vi "MainProgrammer.vi"() -> ()   [LabVIEW 2017]
uses:
  <vilib>/Instr/_visa.llb/Select Event Type.ctl
  <vilib>/Utility/config.llb/Read Key (String).vi
  <vilib>/Utility/config.llb/Write Key (String).vi
  <vilib>/Instr/_visa.llb/VISA Configure Serial Port (Instr).vi
  <vilib>/Utility/config.llb/NI_LVConfig.lvlib
panel:
  out "read buffer":string
  out "Rx":u64
  out "Tx":u64
  in  "stop 7":bool
  in  "stop 6":bool
  out "Error List":string
  out "COM Port":bool
  in  "Flash Baud":u32(ring)=115200 caption="Flash Baudrate" items=["4800"=4800, "9600"=9600, "19200"=19200, "38400"=38400, "57600"=57600, "115200"=115200, "230400"=230400, "460800"=460800, "921600"=921600]
  in  "cmd Baud":u32(ring)=230400 items=["4800"=4800, "9600"=9600, "19200"=19200, "38400"=38400, "57600"=57600, "115200"=115200, "230400"=230400, "460800"=460800, "921600"=921600]
  in  "COM Port":refnum<visa-resource-name>="COM4"
  in  "Next Button":bool
  in  "File Path Control":path
  out "CheckSumArray":u16[][](array[numeric]) format="%.0x"
  out "CheckSum DataB":u16 format="%.0x"
  out "CheckSum Data":u16 format="%.0x"
  out "Array 3":u16[][](array[numeric]) format="%.0x"
  out "Num of Data packet":i32
  out "sumHeader":u16 format="%.0x"
  out "error out":errorcluster
  # "Ver 1.0.5"
  # "© Redler Technologies. All Rights Reserved"
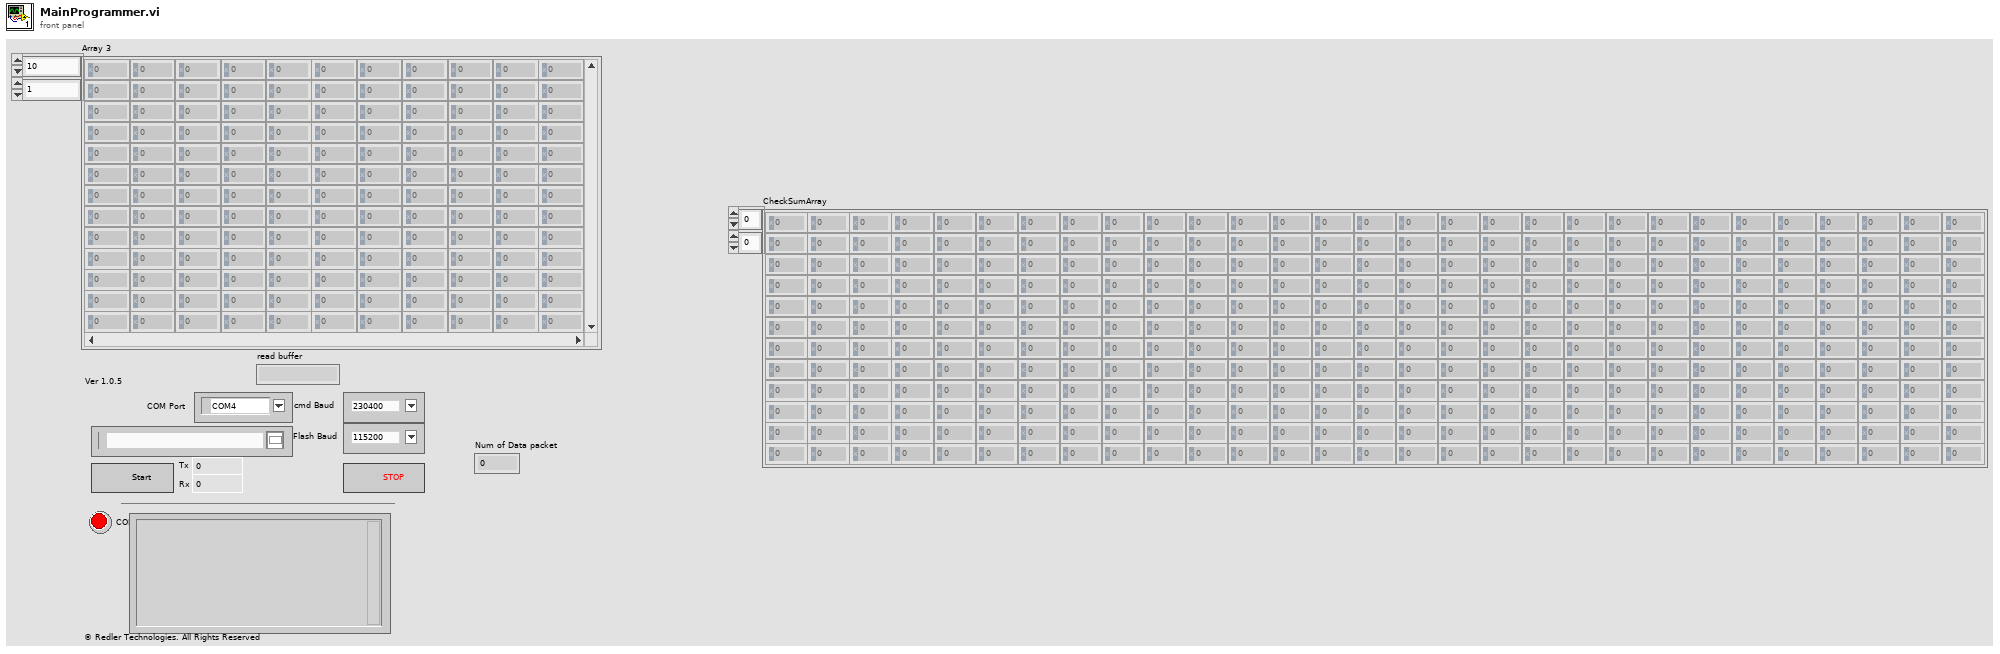
[diagram p1: front panel]
types:
  T1 = typedef "NI_LVConfig.lvlib/Config Data RefNum.ctl" = refnum<k1>
  T2 = cluster{"Send Debug":string, "idx":u16, "DataType":enum8{"Int", " float"}, "Cmd id":u16, "Get/Set":enum8{"Set", "Get"}}
  T3 = cluster{"Data":string, "idx":u16, "DataType":enum8{"Int", " float"}, "Cmd id":u16, "Get/Set":enum8{"Set", "Get"}}
  T4 = typedef "Select Event Type.ctl" = u32
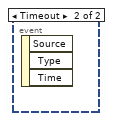
[diagram p3: hidden frame]
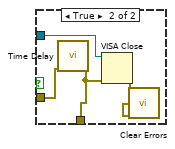
[diagram p4: hidden frame]
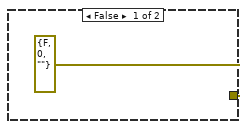
[diagram p5: hidden frame]
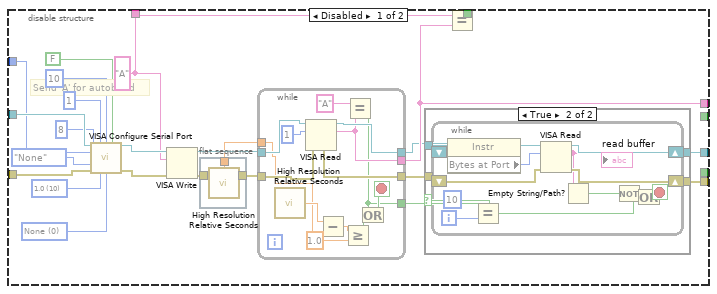
[diagram p7: hidden frame]
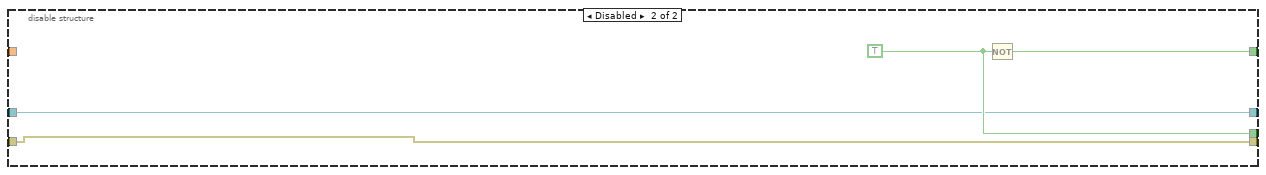
[diagram p10: hidden frame]
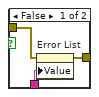
[diagram p13: hidden frame]
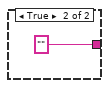
[diagram p16: hidden frame]
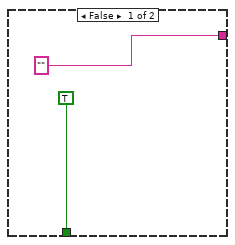
[diagram p17: hidden frame]
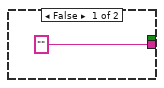
[diagram p18: hidden frame]
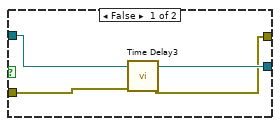
[diagram p19: hidden frame]
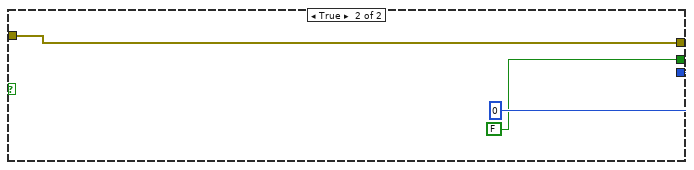
[diagram p20: hidden frame]
diagram:
  w8 = u32 230400 items=["4800"=4800, "9600"=9600, "19200"=19200, "38400"=38400, "57600"=57600, "115200"=115200, "230400"=230400, "460800"=460800, "921600"=921600] ("cmd Baud")
  w9 = u32 230400 items=["4800"=4800, "9600"=9600, "19200"=19200, "38400"=38400, "57600"=57600, "115200"=115200, "230400"=230400, "460800"=460800, "921600"=921600] ("Flash Baud")
  w18 = u32 230400 ("default (0 I32)")
  w3 = "Firmware Path" ("key")
  w4 = "Rayon" ("section")
  n1 = control-ref of="This VI"() -> (w39:refnum<vi>)
  n2 = invoke class="VI" method="Default Vals.Reinit All"(reference=w39, error in=errorcluster {"status"=FALSE, "code"=0, "source"=""} ("error in (no error)")) -> (error out=w7:errorcluster)  [unwired: 1 in, 2 out]
  n3 = property on="Flash Baud" class="Ring (strict)"(error in=w7, "Value"=w9) -> (error out=w10:errorcluster)  [unwired: 1 in, 1 out]
  n4 = property on="cmd Baud" class="Ring (strict)"(error in=w10, "Value"=w8) -> (error out=w6:errorcluster)  [unwired: 1 in, 1 out]
  n5 = call <vilib>:"Application Directory.vi"() -> ("Application Directory"=w37:path)
  n6 = Build Path(base path=w37, name or relative path="data\\RayonSerialProgramerConfigurationFile.ini") -> (appended path=w29:path)
  n7 = call <vilib>:"Open Config Data.vi"("error in (no error)"=w6, "create file if necessary (T)"=FALSE, "configuration file path"=w29) -> ("error out"=w33:errorcluster, "refnum"=w34:T1)  [unwired: 7 out]
  n8 = call-poly <vilib>:"Read Key.vi"("section"=w4, "error in (no error)"=w33, "key"=w3, "refnum"=w34) -> ("error out"=w1:errorcluster, "value"=w32:string, "refnum out"=w5:T1)  [unwired: 2 in, 3 out]
  n9 = String To Path(string=w32) -> (path=w31:path)
  n10 = property on="File Path Control" class="Path"(error in=w1, "Value"=w31) -> (error out=w2:errorcluster)  [unwired: 1 in, 1 out]
  n11 = call-poly <vilib>:"Read Key.vi"("section"=w4, "error in (no error)"=w2, "key"="COM", "refnum"=w5) -> ("error out"=w22:errorcluster, "value"=w14:string, "refnum out"=w27:T1)  [unwired: 2 in, 3 out]
  n12 = Type Cast(type=refnum<visa-resource-name> "COM1" ("UUT COM Port 2"), x=w14) -> (*(type *) &x=w13:refnum<visa-resource-name>)
  n13 = property on="COM Port" class="VISAName"("Value"=w13) -> ()  [unwired: 2 in, 2 out]
  n14 = call-poly <vilib>:"Read Key.vi"("section"=w4, "error in (no error)"=w22, "key"="Flash Baud", "refnum"=w27) -> ("error out"=w21:errorcluster, "value"=w20:string, "refnum out"=w28:T1)  [unwired: 2 in, 3 out]
  n15 = Decimal String To Number(string=w20, default (0L)=w18) -> (number=w16:u32)  [unwired: 1 in, 1 out]
  n16 = property on="Flash Baud" class="Ring (strict)"("Value"=w16) -> ()  [unwired: 2 in, 2 out]
  n17 = call-poly <vilib>:"Read Key.vi"("section"=w4, "error in (no error)"=w21, "key"="Boot Baud", "refnum"=w28) -> ("error out"=w11:errorcluster, "value"=w19:string, "refnum out"=w26:T1)  [unwired: 2 in, 3 out]
  n18 = Decimal String To Number(string=w19, default (0L)=w18) -> (number=w17:u32)  [unwired: 1 in, 1 out]
  n19 = property on="cmd Baud" class="Ring (strict)"("Value"=w17) -> ()  [unwired: 2 in, 2 out]
  n20 = call <vilib>:"Close Config Data.vi"("error in (no error)"=w11, "refnum"=w26) -> ("error out"=w12:errorcluster)  [unwired: 1 in, 8 out]
  n21 = while {
    tunnel: w12 -> [_]
    i -> [w41]
    stop <- w40 stop-if-true
    n22 = event shown="[0] \"stop 7\": Value Change" {
      selector: _ -> [_ _]
      dyn-events: _ -> [_ _]
      timeout: _ -> [_ _]
      tunnel: w41 -> [_ _]
      tunnel: [w42 _] -> w40
      event "stop 7": Value Change {
        n23 = event-data() -> ()  [unwired: 1 in, 3 out]
        n24 = Two Button Dialog(message="Are you sure to close? ", 1:"No" ("F button name (\"Cancel\")"), 2:"Yes" ("T button name (\"OK\")")) -> (T button?=w42:bool)
        n25 = property on="stop 6" class="Bool (strict)"("Value"=w42) -> (error out=w43:errorcluster)  [unwired: 2 in, 1 out]
        n26 = property on="stop 7" class="Bool (strict)"(error in=w43, "Value"=w42) -> (error out=w44:errorcluster)  [unwired: 1 in, 1 out]
        n27 = case shown="True" w42 {
          selector: w42 -> [_ w55]
          tunnel: w44 -> [_ w56]
          frame False {
          }
          frame True {
            w53 = "\r\n"
            n28 = property on="Error List" class="Str"(error in=w56) -> ("Value"=w49:string)  [unwired: 1 in, 2 out]
            n29 = Format Date/Time String(time format string (%c)="%H:%M:%S") -> (date/time string=w52:string)  [unwired: 2 in]
            n30 = Concatenate Strings(w52, " Operation stopped by user") -> (w48:string)
            n31 = Concatenate Strings(w48, w53, w49, w53) -> (w57:string)
            n32 = property on="Error List" class="Str"("Value"=w57) -> (error out=w54:errorcluster)  [unwired: 2 in, 1 out]
            n33 = flat-sequence {
              tunnel: w55 -> [_]
              tunnel: w54 -> [_]
              frame #0 {
                n34 = property on="stop 7" class="Bool (strict)"("Value"=FALSE ("stop 7")) -> ()  [unwired: 2 in, 2 out]
              }
            }
          }
        }
      }
      event Timeout {
        n35 = event-data() -> ()  [unwired: 1 in, 3 out]
      }
    }
  }
  n36 = while {
    tunnel: w12 -> [w67]
    tunnel: w4 -> [w94]
    tunnel: w3 -> [w93]
    tunnel: [w95] -> w30
    tunnel: w29 -> [w92]
    stop <- w62 stop-if-true
    w84 = FALSE ("Next Button")
    n37 = property on="File Path Control" class="Path"(error in=w67, "PTooLngToFt"=enum32{"Abbreviate Path", "Clip Path"}."Abbreviate Path" ("Path Too Long To Fit")) -> (error out=w59:errorcluster)  [unwired: 1 in, 1 out]
    n38 = property on="stop 6" class="Bool (strict)"(error in=w59, "Value"=FALSE ("stop 6")) -> (error out=w74:errorcluster)  [unwired: 1 in, 1 out]
    n39 = while {
      tunnel: ["COM Port"] -> w65
      tunnel: ["Flash Baud"] -> w103
      tunnel: ["cmd Baud"] -> w102
      tunnel: ["File Path Control"] -> w77
      tunnel: w94 -> [w984]
      tunnel: w74 -> [w980]
      tunnel: w93 -> [w982]
      tunnel: w92 -> [w978]
      tunnel: [w970] -> w66
      stop <- w981 stop-if-true
      n40 = call <vilib>:"Open Config Data.vi"("error in (no error)"=w980, "create file if necessary (T)"=FALSE, "configuration file path"=w978) -> ("error out"=w979:errorcluster, "refnum"=w976:T1)  [unwired: 7 out]
      n41 = Path To String(path="File Path Control") -> (string=w983:string)
      n42 = call <vilib>:"Is Path and Not Empty.vi"("path"="File Path Control") -> ("Is Path and Not Empty?"=w987:bool)  [unwired: 4 in]
      n43 = Not(x=w987) -> (.not. x?=w985:bool)
      n44 = And(x=w985, y="Next Button") -> (x .and. y?=w986:bool)
      n45 = case shown="False" w986 {
        tunnel: w984 -> [w996 _]
        tunnel: w979 -> [w1013 w1014]
        tunnel: w983 -> [w1012 _]
        tunnel: w982 -> [w1011 _]
        tunnel: w976 -> [w1010 _]
        tunnel: [w1009 w1015] -> w970
        tunnel: "COM Port" -> [w993 _]
        tunnel: "Flash Baud" -> [w990 _]
        tunnel: "cmd Baud" -> [w992 _]
        frame False {
          n46 = call-poly <vilib>:"Write Key.vi"("section"=w996, "error in (no error)"=w1013, "value"=w1012, "key"=w1011, "refnum"=w1010) -> ("error out"=w1003:errorcluster, "refnum out"=w999:T1)  [unwired: 1 in, 4 out]
          n47 = Type Cast(type="", x=w993) -> (*(type *) &x=w991:string)
          n48 = call-poly <vilib>:"Write Key.vi"("section"=w996, "error in (no error)"=w1003, "value"=w991, "key"="COM", "refnum"=w999) -> ("error out"=w1002:errorcluster, "refnum out"=w998:T1)  [unwired: 1 in, 4 out]
          n49 = Number To Decimal String(number=w990) -> (decimal integer string=w1008:string)  [unwired: 1 in]
          n50 = call-poly <vilib>:"Write Key.vi"("section"=w996, "error in (no error)"=w1002, "value"=w1008, "key"="Flash Baud", "refnum"=w998) -> ("error out"=w1001:errorcluster, "refnum out"=w997:T1)  [unwired: 1 in, 4 out]
          n51 = Number To Decimal String(number=w992) -> (decimal integer string=w1005:string)  [unwired: 1 in]
          n52 = call-poly <vilib>:"Write Key.vi"("section"=w996, "error in (no error)"=w1001, "value"=w1005, "key"="Boot Baud", "refnum"=w997) -> ("error out"=w1000:errorcluster, "refnum out"=w995:T1)  [unwired: 1 in, 4 out]
          n53 = call <vilib>:"Close Config Data.vi"("error in (no error)"=w1000, "refnum"=w995) -> ("error out"=w1009:errorcluster)  [unwired: 1 in, 8 out]
        }
        frame True {
          n54 = One Button Dialog(message="Please select a valid path !") -> ()  [unwired: 1 in, 1 out]
          n55 = property on="Next Button" class="Bool (strict)"(error in=w1014, "Value"=FALSE ("Next Button")) -> (error out=w1015:errorcluster)  [unwired: 1 in, 1 out]
        }
      }
      n56 = property on="Next Button" class="Bool (strict)"("Blinking"="Next Button") -> ()  [unwired: 2 in, 2 out]
      n57 = And(x="Next Button", y=w987) -> (x .and. y?=w988:bool)
      n58 = Or(x=w988, y=FALSE) -> (x .or. y?=w981:bool)
    }
    n59 = VISA Flush I/O Buffer(VISA resource name=w65, error in (no error)=w66) -> (VISA resource name out=w63:refnum<visa-resource-name>, error out=w64:errorcluster)  [unwired: 1 in]
    n60 = flat-sequence {
      tunnel: [w121] -> w73
      tunnel: " Openning COM Port..." -> [w120]
      tunnel: w69 -> [_]
      frame #0 {
        n61 = Format Date/Time String(time format string (%c)="%H:%M:%S") -> (date/time string=w119:string)  [unwired: 2 in]
        n62 = Concatenate Strings(w119, w120) -> (w121:string)
      }
    }
    n63 = call <vilib>:"Clear Errors.vi"("error in (no error)"=w64) -> ("error out"=w91:errorcluster)  [unwired: 5 in, 1 out]
    n64 = property on="Error List" class="Str"(error in=w91, "Value"="") -> (error out=w69:errorcluster)  [unwired: 1 in, 1 out]
    n65 = Concatenate Strings("\r\n", w73) -> (w99:string)
    n66 = flat-sequence {
      tunnel: [w107] -> w71
      tunnel: [w105] -> w70
      tunnel: w98 -> [_]
      frame #0 {
        n67 = Format Date/Time String(time format string (%c)="%H:%M:%S") -> (date/time string=w112:string)  [unwired: 2 in]
        n68 = Format Date/Time String(time format string (%c)="%H:%M:%S") -> (date/time string=w115:string)  [unwired: 2 in]
        n69 = Format Date/Time String(time format string (%c)="%H:%M:%S") -> (date/time string=w117:string)  [unwired: 2 in]
        n70 = Concatenate Strings(w112, " Openning COM Port success !") -> (w105:string)
        n71 = Concatenate Strings(w115, " Openning COM Port failed !") -> (w108:string)
        n72 = Concatenate Strings(w117, " Check COM adaptor." ("string"), "\r\n") -> (w109:string)
        n73 = Concatenate Strings(w109, w108) -> (w107:string)
      }
    }
    n74 = property on="Error List" class="Str"(error in=w69, "Value"=w99) -> (error out=w98:errorcluster)  [unwired: 1 in, 1 out]
    n75 = call <vilib>:"Clear Errors.vi"("error in (no error)"=w98) -> ("error out"=w87:errorcluster)  [unwired: 5 in, 1 out]
    n76 = Unbundle By Name(w98) -> ("status"=w80:bool)
    n77 = call "ConvertDataFrom File (SubVI).vi"("File Path Control"=w77) -> ("WrongFile?"=w75:bool, "Full Text File"=w79:u8[], "Header"=w78:u16[])  [unwired: 13 in, 3 out]
    n78 = Select(t=w71, s=w80, f=w70) -> (s? t:f=w89:string)
    n79 = property on="Error List" class="Str"(error in=w87) -> (error out=w82:errorcluster, "Value"=w97:string)  [unwired: 1 in, 1 out]
    n80 = case shown="False" w80 {
      tunnel: w82 -> [w122 w126]
      tunnel: [w122 w125] -> w81
      tunnel: w63 -> [_ w124]
      frame False {
      }
      frame True {
        n81 = call "Time Delay"("error in (no error)"=w126) -> ("error out"=w125:errorcluster)  [unwired: 10 in]
        n82 = VISA Close(VISA resource name=w124, error in (no error)=w125) -> (error out=w123:errorcluster)
        n83 = call <vilib>:"Clear Errors.vi"("error in (no error)"=w123) -> ()  [unwired: 5 in, 2 out]
      }
    }
    n84 = Not(x=w80) -> (.not. x?=w60:bool)
    n85 = Concatenate Strings(w89, w97) -> (w101:string)
    n86 = property on="Error List" class="Str"(error in=w81, "Value"=w101) -> (error out=w100:errorcluster)  [unwired: 1 in, 1 out]
    n87 = And(x=w75, y=w60) -> (x .and. y?=w76:bool)
    n88 = case shown="True" w76 {
      tunnel: w103 -> [_ w215]
      tunnel: w102 -> [_ w214]
      tunnel: w100 -> [_ w205]
      tunnel: w63 -> [_ w204]
      tunnel: [errorcluster {"status"=FALSE, "code"=0, "source"=""} ("error out") w170] -> w96
      tunnel: w79 -> [_ w173]
      tunnel: w78 -> [_ w172]
      frame False {
      }
      frame True {
        (unwired) "uRayonM1_1.05.01_HW2.txt" ("name or relative path")
        (unwired) u16[] [1536, 15872, 128, 15912, 0, 37503, 63861, 36326, 15872] ("Array 4")
        # "Receive header checksum from the UUT"
        # "- U16 array to be send in string\n- Perform the header checksum"
        n89 = case shown="False" FALSE {
          tunnel: w205 -> [w537 w563]
          tunnel: w204 -> [_ w569]
          tunnel: [w533 w565] -> w203
          tunnel: [w537 w566] -> w190
          tunnel: [w534 w568] -> w197
          tunnel: [TRUE w567] -> w171
          tunnel: [FALSE ("Value") w554] -> w134
          tunnel: u8[] [73, 93, 62, 64, 16, 81, 192] ("output array") -> [_ w553]
          frame False {
            n90 = while {
              tunnel: [w544] -> w534
              tunnel: [w543] -> w533
              i -> [w540]
              stop <- w541 stop-if-true
              n91 = control-ref of="Tx"() -> (w550:refnum<vi>)
              n92 = control-ref of="Rx"() -> (w551:refnum<vi>)
              n93 = call "Connect COM Port & AutoBaud (SubVI).vi"("Rx"=w551, "Tx"=w550) -> ("Success?"=w542:bool, "VISA Refnum out"=w549:refnum<visa-resource-name>)  [unwired: 7 in, 1 out]
              "COM Port" <- w542
              n94 = Equal?(x=10, y=w540) -> (x = y?=w539:bool)
              n95 = call "TxRx SingleBoard (SubVI).vi"("VISA Refnum in"=w549, "DataMessage Tx"=T2 {"Send Debug"="0", "idx"=1, "DataType"=enum."Int", "Cmd id"=62, "Get/Set"=enum."Get"}, "Tx"=w550, "Rx"=w551) -> ("VISA Refnum out"=w543:refnum<visa-resource-name>, "RxMessage"=w548:u8[], "error out"=w552:errorcluster)  [unwired: 9 in, 4 out]
              n96 = Or(x=w542, y=w539) -> (x .or. y?=w541:bool)
              n97 = call "DescriptReceivedMsg SingleBoard (SubVI).vi"("error constant"=w552, "RxMessageArray"=w548) -> ("DataMessage Rx"=w547:T3)  [unwired: 8 in, 1 out]
              n98 = Unbundle By Name(w547) -> ("Data"=w545:string)
              n99 = Decimal String To Number(string=w545) -> (number=w544:i32)  [unwired: 2 in, 1 out]
            }
          }
          frame True {
            w559 = "\r\n"
            w580 = u16 0 items=["None", "XON/XOFF", "RTS/CTS", "XON/XOFF & RTS/CTS", "DTR/DSR", "XON/XOFF & DTR/DSR"] ("flow control (0:none)")
            w579 = u16 10 items=["1.0"=10, "1.5"=15, "2.0"=20] ("stop bits (10: 1 bit)")
            w581 = T4 1073684533 items=["Service Request"=1073684491, "Trigger"=3221168138, "Clear"=1073684493, "VXI Signal"=1073684512, "VXI/VME Interrupt"=3221168161, "VXI/VME Sysfail"=1073684509, "VXI/VME Sysreset"=1073684510, "GPIB CIC"=1073684498, "GPIB Talk"=1073684499, "GPIB Listen"=1073684500, "PXI Interrupt"=1073684514, "Serial Break"=1073684515, "Serial TermChar"=1073684516, "Serial CTS"=1073684521, "Serial DSR"=1073684522, "Serial DCD"=1073684524, "Serial RI"=1073684526, "Serial Character"=1073684533, "USB Interrupt"=1073684535, "All Enabled"=1073709055] ("Event Type")
            n100 = property on="Error List" class="Str"(error in=w563) -> (error out=w562:errorcluster, "Value"=w560:string)  [unwired: 1 in, 1 out]
            n101 = Format Date/Time String(time format string (%c)="%H:%M:%S") -> (date/time string=w557:string)  [unwired: 2 in]
            n102 = Concatenate Strings(w557, " Getting Driver version...") -> (w555:string)
            n103 = Concatenate Strings(w555, w559, w560, w559) -> (w564:string)
            n104 = property on="Error List" class="Str"(error in=w562, "Value"=w564) -> (error out=w561:errorcluster)  [unwired: 1 in, 1 out]
            n105 = call-poly "VISA Configure Serial Port"("VISA resource name"=w569, "timeout (10sec)"=u32 200, "Enable Termination\nChar (T)"=FALSE ("Enable Termination\nChar (T)"), "baud rate (9600)"=u32 460800, "data bits (8)"=u16 8, "parity (0:none)"=enum16{"None", "Odd", "Even", "Mark", "Space"}."None", "error in (no error)"=w561, "stop bits (10: 1 bit)"=w579, "flow control (0:none)"=w580) -> ("VISA resource name out"=w573:refnum<visa-resource-name>, "error out"=w574:errorcluster)  [unwired: 5 in]
            n106 = VISA Enable Event(8:w574, 10:w581, 11:w573) -> (0:w571:errorcluster, 3:w572:refnum<visa-resource-name>)  [unwired: 1 in]
            n107 = Byte Array To String(unsigned byte array=w553) -> (string=w585:string)
            n108 = VISA Write(VISA resource name=w572, write buffer=w585, error in (no error)=w571) -> (VISA resource name out=w586:refnum<visa-resource-name>, error out=w584:errorcluster)  [unwired: 1 out]
            n109 = flat-sequence {
              tunnel: w584 -> [w588]
              tunnel: [w588] -> w583
              tunnel: [w587] -> w582
              frame #0 {
                n110 = call <vilib>:"High Resolution Relative Seconds.vi"() -> ("relative seconds"=w587:dbl)
              }
            }
            n111 = while {
              tunnel: w583 -> [w606]
              tunnel: [w603] -> w566
              tunnel: w586 -> [w605]
              tunnel: [w604] -> w565
              tunnel: w582 -> [w596]
              tunnel: [w591] -> w568
              tunnel: [w590] -> w567
              tunnel: [w589] -> w554
              stop <- w593 stop-if-true
              n112 = call <vilib>:"High Resolution Relative Seconds.vi"() -> ("relative seconds"=w597:dbl)
              n113 = VISA Read(VISA resource name=w605, byte count=u32 11, error in (no error)=w606) -> (VISA resource name out=w604:refnum<visa-resource-name>, read buffer=w601:string, return count=w598:u32, error out=w603:errorcluster)
              n114 = Subtract(x=w597, y=w596) -> (x-y=w594:dbl)
              n115 = String To Byte Array(string=w601) -> (unsigned byte array=w600:u8[])
              n116 = Not Equal To 0?(x=w598) -> (x != 0?=w590:bool)
              n117 = Greater Or Equal?(x=w594, y=3.0) -> (x >= y?=w592:bool)
              n118 = call "Data_Convert.vi"("Data Type"=u8 0, "Array"=w600) -> ("D Int out"=w591:i32)  [unwired: 2 out]
              n119 = property on="stop 6" class="Bool (strict)"() -> ("Value"=w589:bool)  [unwired: 2 in, 2 out]
              n120 = Compound Arithmetic op=OR(w589, w590, w592) -> (w593:bool)
            }
          }
        }
        n121 = flat-sequence {
          tunnel: [w409] -> w152
          tunnel: [w405] -> w151
          tunnel: [w403] -> w150
          tunnel: [w401] -> w149
          tunnel: [" Sending autobaud operation..." ("string")] -> w148
          tunnel: [" Getting Driver version failed !" ("f")] -> w147
          tunnel: ["\r\n"] -> w146
          tunnel: w142 -> [_]
          frame #0 {
            n122 = Format Date/Time String(time format string (%c)="%H:%M:%S") -> (date/time string=w411:string)  [unwired: 2 in]
            n123 = Format Date/Time String(time format string (%c)="%H:%M:%S") -> (date/time string=w407:string)  [unwired: 2 in]
            n124 = Format Date/Time String(time format string (%c)="%H:%M:%S") -> (date/time string=w401:string)  [unwired: 2 in]
            n125 = Format Date/Time String(time format string (%c)="%H:%M:%S") -> (date/time string=w403:string)  [unwired: 2 in]
            n126 = Concatenate Strings(w411, " Driver Version: " ("string")) -> (w409:string)
            n127 = Concatenate Strings(w407, " Sending autobaud operation...") -> (w405:string)
          }
        }
        n128 = Concatenate Strings(w149, w147) -> (w144:string)
        n129 = Concatenate Strings(w150, w148, w146) -> (w145:string)
        n130 = call <vilib>:"Clear Errors.vi"("error in (no error)"=w190) -> ("error out"=w181:errorcluster)  [unwired: 5 in, 1 out]
        n131 = Format Into String(w197) -> (resulting string=w153:string)  [unwired: 3 in, 1 out]
        n132 = Concatenate Strings(w145, w144) -> (w143:string)
        n133 = property on="Error List" class="Str"(error in=w181) -> (error out=w142:errorcluster, "Value"=w155:string)  [unwired: 1 in, 1 out]
        n134 = Concatenate Strings(w151, "\r\n", w152, w153) -> (w179:string)
        n135 = Select(t=w179, s=w171, f=w143) -> (s? t:f=w168:string)
        n136 = Concatenate Strings(w168, "\r\n", w155) -> (w198:string)
        n137 = case shown="False" w134 {
          tunnel: w198 -> [w376 _]
          tunnel: [w375 w377] -> w196
          tunnel: w142 -> [w374 w377]
          frame False {
            n138 = property on="Error List" class="Str"(error in=w374, "Value"=w376) -> (error out=w375:errorcluster)  [unwired: 1 in, 1 out]
          }
          frame True {
          }
        }
        n139 = disable-structure shown="Disabled" {
          disable-tunnel: [w233 w244] -> w217
          disable-tunnel: w214 -> [w232 _]
          disable-tunnel: [w231 w245] -> w213
          disable-tunnel: w203 -> [w230 w244]
          disable-tunnel: w196 -> [w229 w245]
          frame Disabled {
            w235 = u16 0 items=["None", "LastBit", "TermChar", "Break"] ("Serial Settings:Serial End Mode for Writes")
            w238 = u16 0 items=["None", "XON/XOFF", "RTS/CTS", "XON/XOFF & RTS/CTS", "DTR/DSR", "XON/XOFF & DTR/DSR"] ("flow control (0:none)")
            w239 = u16 10 items=["1.0"=10, "1.5"=15, "2.0"=20] ("stop bits (10: 1 bit)")
            n140 = call <vilib>:"Clear Errors.vi"("error in (no error)"=w229) -> ("error out"=w228:errorcluster)  [unwired: 5 in, 1 out]
            n141 = call-poly "VISA Configure Serial Port"("VISA resource name"=w230, "timeout (10sec)"=u32 200, "termination char\n(0xA = '\\n' = LF)"=u8 10 ("termination char\n(0xA = '\\n' = LF)"), "Enable Termination\nChar (T)"=FALSE ("Enable Termination\nChar (T)"), "baud rate (9600)"=w232, "data bits (8)"=u16 8, "parity (0:none)"=enum16{"None", "Odd", "Even", "Mark", "Space"}."None", "error in (no error)"=w228, "stop bits (10: 1 bit)"=w239, "flow control (0:none)"=w238) -> ("VISA resource name out"=w236:refnum<visa-resource-name>, "error out"=w237:errorcluster)  [unwired: 4 in]
            n142 = property class="Instr"(reference=w236, error in=w237, "Serial Settings:End Mode for Writes"=w235, "Message Based Settings:Send End Enable"=FALSE) -> (reference out=w233:refnum<visa-resource-name>, error out=w231:errorcluster)
          }
          frame Enabled {
          }
        }
        n143 = flat-sequence {
          tunnel: w213 -> [w608]
          tunnel: [w608] -> w212
          tunnel: [w607] -> w211
          frame #0 {
            n144 = call <vilib>:"High Resolution Relative Seconds.vi"() -> ("relative seconds"=w607:dbl)
          }
        }
        n145 = disable-structure shown="Enabled" {
          disable-tunnel: [w255 w355] -> w226
          disable-tunnel: w217 -> [w254 w355]
          disable-tunnel: w215 -> [w253 _]
          disable-tunnel: w212 -> [w252 w354]
          disable-tunnel: w211 -> [w251 _]
          disable-tunnel: [w247 w356] -> w210
          disable-tunnel: [w250 w354] -> w189
          disable-tunnel: [w249 _] -> w178
          disable-tunnel: w171 -> [w248 _]
          disable-tunnel: [w246 w357] -> w130
          frame Enabled {
            n146 = while {
              tunnel: [w266] -> w257
              tunnel: [w262] -> w256
              tunnel: w253 -> [w272]
              tunnel: w251 -> [w270]
              tunnel: w252 -> [w280]
              tunnel: [w260] -> w250
              tunnel: w254 -> [w281]
              tunnel: [w261] -> w255
              tunnel: [w267] -> _
              tunnel: [w265] -> w249
              tunnel: w248 -> [_]
              tunnel: [w263] -> w246
              tunnel: [w259] -> _
              tunnel: [w258] -> w247
              i -> [w275]
              stop <- w278 stop-if-true
              # "Send cmd for bootloader enable"
              n147 = case shown="True" TRUE {
                tunnel: w281 -> [w346 w353]
                tunnel: w280 -> [w345 w352]
                tunnel: [w346 w351] -> w273
                tunnel: [w345 w347] -> w274
                tunnel: u8[] [73, 93, 65, 0, 0, 1, 0, 0, 0, 80, 248] ("output array") -> [_ w349]
                frame False {
                }
                frame True {
                  n148 = Byte Array To String(unsigned byte array=w349) -> (string=w348:string)
                  n149 = VISA Write(VISA resource name=w353, write buffer=w348, error in (no error)=w352) -> (VISA resource name out=w351:refnum<visa-resource-name>, error out=w350:errorcluster)  [unwired: 1 out]
                  n150 = call "Time Delay2"("error in (no error)"=w350) -> ("error out"=w347:errorcluster)  [unwired: 10 in]
                }
              }
              n151 = call <vilib>:"High Resolution Relative Seconds.vi"() -> ("relative seconds"=w271:dbl)
              n152 = Subtract(x=w271, y=w270) -> (x-y=w269:dbl)
              n153 = Greater Or Equal?(x=w269, y=3.0) -> (x >= y?=w267:bool)
              n154 = disable-structure shown="Enabled" {
                disable-tunnel: w274 -> [w302 w342]
                disable-tunnel: w273 -> [w301 w343]
                disable-tunnel: w272 -> [w300 _]
                disable-tunnel: [w299 "A" ("x")] -> w266
                disable-tunnel: [w295 w340] -> w265
                disable-tunnel: [w294 _] -> w262
                disable-tunnel: [w285 w343] -> w261
                disable-tunnel: [w283 w344] -> w260
                disable-tunnel: [_ w340] -> w259
                disable-tunnel: [_ w340] -> w258
                frame Disabled {
                  w287 = u16 0 items=["None", "XON/XOFF", "RTS/CTS", "XON/XOFF & RTS/CTS", "DTR/DSR", "XON/XOFF & DTR/DSR"] ("flow control (0:none)")
                  w288 = u16 10 items=["1.0"=10, "1.5"=15, "2.0"=20] ("stop bits (10: 1 bit)")
                  w294 = "A" ("write buffer")
                  # "Send 'A' for autobaud"
                  n155 = call-poly "VISA Configure Serial Port"("VISA resource name"=w301, "timeout (10sec)"=u32 1, "termination char\n(0xA = '\\n' = LF)"=u8 10 ("termination char\n(0xA = '\\n' = LF)"), "Enable Termination\nChar (T)"=FALSE ("Enable Termination\nChar (T)"), "baud rate (9600)"=w300, "data bits (8)"=u16 8, "parity (0:none)"=enum16{"None", "Odd", "Even", "Mark", "Space"}."None", "error in (no error)"=w302, "stop bits (10: 1 bit)"=w288, "flow control (0:none)"=w287) -> ("VISA resource name out"=w303:refnum<visa-resource-name>, "error out"=w304:errorcluster)  [unwired: 4 in]
                  n156 = VISA Write(VISA resource name=w303, write buffer=w294, error in (no error)=w304) -> (VISA resource name out=w305:refnum<visa-resource-name>, error out=w298:errorcluster)  [unwired: 1 out]
                  n157 = flat-sequence {
                    tunnel: w298 -> [w325]
                    tunnel: [w325] -> w297
                    tunnel: [w324] -> w296
                    frame #0 {
                      n158 = call <vilib>:"High Resolution Relative Seconds.vi"() -> ("relative seconds"=w324:dbl)
                    }
                  }
                  n159 = while {
                    tunnel: [w335] -> w299
                    tunnel: w296 -> [w330]
                    tunnel: w297 -> [w336]
                    tunnel: [w332] -> w282
                    tunnel: w305 -> [w337]
                    tunnel: [w339] -> w286
                    tunnel: [w326] -> w284
                    stop <- w333 stop-if-true
                    n160 = call <vilib>:"High Resolution Relative Seconds.vi"() -> ("relative seconds"=w331:dbl)
                    n161 = VISA Read(VISA resource name=w337, byte count=u32 1, error in (no error)=w336) -> (VISA resource name out=w339:refnum<visa-resource-name>, read buffer=w335:string, error out=w332:errorcluster)  [unwired: 1 out]
                    n162 = Subtract(x=w331, y=w330) -> (x-y=w329:dbl)
                    n163 = Greater Or Equal?(x=w329, y=1.0) -> (x >= y?=w328:bool)
                    n164 = Equal?(x="A", y=w335) -> (x = y?=w326:bool)
                    n165 = Or(x=w326, y=w328) -> (x .or. y?=w333:bool)
                  }
                  n166 = case shown="True" w284 {
                    tunnel: w286 -> [w307 w308]
                    tunnel: [w307 w311] -> w285
                    tunnel: [w306 w310] -> w283
                    tunnel: w282 -> [w306 w309]
                    frame False {
                    }
                    frame True {
                      n167 = while {
                        shift-right: [w322] -> w310
                        shift-left: w309 -> [w321]
                        shift-right: [w323] -> w311
                        shift-left: w308 -> [w320]
                        i -> [w315]
                        stop <- w313 stop-if-true
                        n168 = property class="Instr"(reference=w320) -> ("Bytes at Port"=w319:u32)  [unwired: 1 in, 2 out]
                        n169 = Equal?(x=10, y=w315) -> (x = y?=w312:bool)
                        n170 = VISA Read(VISA resource name=w320, byte count=w319, error in (no error)=w321) -> (VISA resource name out=w323:refnum<visa-resource-name>, read buffer=w318:string, error out=w322:errorcluster)  [unwired: 1 out]
                        "read buffer" <- w318
                        n171 = Empty String/Path?(string/path=w318) -> (empty?=w317:bool)
                        n172 = Not(x=w317) -> (.not. x?=w316:bool)
                        n173 = Or(x=w316, y=w312) -> (x .or. y?=w313:bool)
                      }
                    }
                  }
                  n174 = Equal?(x=w294, y=w299) -> (x = y?=w295:bool)
                }
                frame Enabled {
                  n175 = call "BootLoader AutoBaud (SubVI).vi"("VISA"=w343, "error in (no error)"=w342) -> ("error out"=w344:errorcluster, "Success?"=w340:bool)  [unwired: 8 in]
                }
              }
              n176 = property on="stop 6" class="Bool (strict)"() -> ("Value"=w263:bool)  [unwired: 2 in, 2 out]
              n177 = Equal?(x=10, y=w275) -> (x = y?=w276:bool)
              n178 = Compound Arithmetic op=OR(w265, w276, w263) -> (w278:bool)
            }
            n179 = Equal?(x=w256, y=w257) -> ()  [unwired: 1 out]
          }
          frame Disabled {
            w356 = TRUE ("x")
            n180 = Not(x=w356) -> (.not. x?=w357:bool)
          }
        }
        n181 = call <vilib>:"Application Directory.vi"() -> ("Application Directory"=w223:path)
        n182 = Build Path(base path=w223, name or relative path="uRayonM1_1.03.02.txt") -> ()  [unwired: 1 out]
        n183 = flat-sequence {
          tunnel: [w384] -> w141
          tunnel: [w378] -> w140
          tunnel: w139 -> [_]
          frame #0 {
            n184 = Format Date/Time String(time format string (%c)="%H:%M:%S ") -> (date/time string=w393:string)  [unwired: 2 in]
            n185 = Format Date/Time String(time format string (%c)="%H:%M:%S ") -> (date/time string=w392:string)  [unwired: 2 in]
            n186 = Format Date/Time String(time format string (%c)="%H:%M:%S ") -> (date/time string=w391:string)  [unwired: 2 in]
            n187 = Format Date/Time String(time format string (%c)="%H:%M:%S ") -> (date/time string=w390:string)  [unwired: 2 in]
            n188 = Concatenate Strings(w393, "Erase start..." ("string"), "\r\n") -> (w380:string)
            n189 = Concatenate Strings(w392, "Autobaud handshake success !") -> (w379:string)
            n190 = Concatenate Strings(w391, "Try changing baudrate, verify COM adaptor, Power Supply and reset unit.", "\r\n") -> (w386:string)
            n191 = Concatenate Strings(w390, "No response, autobaud handshake failed !" ("string")) -> (w385:string)
            n192 = Concatenate Strings(w380, w379) -> (w378:string)
            n193 = Concatenate Strings(w386, w385) -> (w384:string)
          }
        }
        n194 = Select(t=w140, s=w178, f=w141) -> (s? t:f=w167:string)
        n195 = call <vilib>:"Clear Errors.vi"("error in (no error)"=w189) -> ("error out"=w186:errorcluster)  [unwired: 5 in, 1 out]
        n196 = property on="Error List" class="Str"(error in=w186) -> (error out=w139:errorcluster, "Value"=w157:string)  [unwired: 1 in, 1 out]
        n197 = Concatenate Strings(w167, "\r\n", w157) -> (w202:string)
        n198 = case shown="False" w130 {
          tunnel: w202 -> [w372 _]
          tunnel: [w371 w373] -> w129
          tunnel: w139 -> [w370 w373]
          frame False {
            n199 = property on="Error List" class="Str"(error in=w370, "Value"=w372) -> (error out=w371:errorcluster)  [unwired: 1 in, 1 out]
          }
          frame True {
          }
        }
        n200 = flat-sequence {
          tunnel: w129 -> [w951]
          tunnel: [w956] -> w225
          tunnel: [w953] -> w224
          tunnel: w172 -> [w952]
          tunnel: [w951] -> w218
          frame #0 {
            (unwired) u16[] [43528, 0, 0, 0, 0, 0, 0, 0, 0, 15872, 36326]
            n201 = for {
              tunnel: w952 -> [w969] mode=indexing
              shift-right: [w964] -> w956
              shift-left: u8[] [] -> [w963]
              shift-right: [w961] -> w955
              shift-left: u16 0 -> [w962]
              i -> [w968]
              n202 = Split Number(x=w969) -> (hi(x)=w960:u8, lo(x)=w959:u8)
              n203 = Build Array(w960, w959) -> (w966:u8[])
              n204 = Compound Arithmetic op=ADD(w962, w960, w959) -> (w961:u16)
              n205 = Multiply(x=w968, y=2) -> (x*y=w965:i32)
              n206 = Insert Into Array(array=w963, index=w965, new element=w966) -> (w964:u8[])
            }
            "sumHeader" <- w955
            n207 = Type Cast(type="", x=w955) -> (*(type *) &x=w953:string)
          }
        }
        n208 = And(x=w210, y=TRUE) -> (x .and. y?=w209:bool)
        n209 = case shown="True" w209 {
          tunnel: w218 -> [w894 w900]
          tunnel: w226 -> [w895 w901]
          tunnel: [w894 w913] -> w188
          tunnel: [w895 w912] -> w219
          tunnel: w225 -> [_ w897]
          tunnel: ["0" ("read buffer") w911] -> w222
          tunnel: ["0" ("read buffer") w910] -> w221
          tunnel: [TRUE w902] -> _
          frame False {
          }
          frame True {
            (unwired) "ª\b" ("write buffer")
            n210 = Byte Array To String(unsigned byte array=w897) -> (string=w896:string)
            n211 = VISA Write(VISA resource name=w901, write buffer=w896, error in (no error)=w900) -> (VISA resource name out=w898:refnum<visa-resource-name>, error out=w899:errorcluster)  [unwired: 1 out]
            n212 = flat-sequence {
              tunnel: w899 -> [w918]
              tunnel: [w918] -> w909
              tunnel: [w917] -> w908
              frame #0 {
                n213 = call <vilib>:"High Resolution Relative Seconds.vi"() -> ("relative seconds"=w917:dbl)
              }
            }
            n214 = while {
              tunnel: w898 -> [w947]
              tunnel: [w948] -> w914
              tunnel: w909 -> [w946]
              tunnel: [w949] -> w907
              tunnel: [w941] -> w910
              tunnel: w908 -> [w937]
              tunnel: [w935] -> w903
              stop <- w943 stop-if-true
              n215 = VISA Read(VISA resource name=w947, byte count=u32 1, error in (no error)=w946) -> (VISA resource name out=w948:refnum<visa-resource-name>, read buffer=w941:string, return count=w942:u32, error out=w949:errorcluster)
              n216 = call <vilib>:"High Resolution Relative Seconds.vi"() -> ("relative seconds"=w938:dbl)
              n217 = Not Equal?(x=w942, y=u32 0) -> (x != y?=w944:bool)
              n218 = Subtract(x=w938, y=w937) -> (x-y=w939:dbl)
              n219 = property on="stop 6" class="Bool (strict)"() -> ("Value"=w936:bool)  [unwired: 2 in, 2 out]
              n220 = Greater Or Equal?(x=w939, y=10.0) -> (x >= y?=w935:bool)
              n221 = Compound Arithmetic op=OR(w944, w936, w935) -> (w943:bool)
              n222 = property on="stop 6" class="Bool (strict)"("Value"=w935) -> ()  [unwired: 2 in, 2 out]
            }
            n223 = flat-sequence {
              tunnel: w907 -> [w915]
              tunnel: [w916] -> w905
              tunnel: [w915] -> w906
              frame #0 {
                n224 = call <vilib>:"High Resolution Relative Seconds.vi"() -> ("relative seconds"=w916:dbl)
              }
            }
            n225 = while {
              tunnel: w914 -> [w933]
              tunnel: [w930] -> w912
              tunnel: w906 -> [w934]
              tunnel: [w931] -> w913
              tunnel: [w925] -> w911
              tunnel: w905 -> [w921]
              tunnel: [w920] -> w904
              stop <- w926 stop-if-true
              n226 = VISA Read(VISA resource name=w933, byte count=u32 1, error in (no error)=w934) -> (VISA resource name out=w930:refnum<visa-resource-name>, read buffer=w925:string, return count=w927:u32, error out=w931:errorcluster)
              n227 = call <vilib>:"High Resolution Relative Seconds.vi"() -> ("relative seconds"=w924:dbl)
              n228 = Not Equal?(x=w927, y=u32 0) -> (x != y?=w929:bool)
              n229 = Subtract(x=w924, y=w921) -> (x-y=w923:dbl)
              n230 = property on="stop 6" class="Bool (strict)"() -> ("Value"=w919:bool)  [unwired: 2 in, 2 out]
              n231 = Greater Or Equal?(x=w923, y=10.0) -> (x >= y?=w920:bool)
              n232 = Compound Arithmetic op=OR(w929, w919, w920) -> (w926:bool)
            }
            n233 = Or(x=w904, y=w903) -> (x .or. y?=w902:bool)
          }
        }
        n234 = call <vilib>:"Clear Errors.vi"("error in (no error)"=w188) -> ("error out"=w180:errorcluster)  [unwired: 5 in, 1 out]
        n235 = property on="Error List" class="Str"(error in=w180) -> (error out=w138:errorcluster, "Value"=w159:string)  [unwired: 1 in, 1 out]
        n236 = Concatenate Strings(w222, w221) -> (w220:string)
        n237 = Equal?(x=w224, y=w220) -> (x = y?=w175:bool)
        n238 = case shown="True" w178 {
          tunnel: w175 -> [_ w459]
          tunnel: ["" w458] -> w166
          tunnel: w138 -> [_ w455]
          frame False {
          }
          frame True {
            n239 = flat-sequence {
              tunnel: [w466] -> w456
              tunnel: [w460] -> w457
              tunnel: w455 -> [_]
              frame #0 {
                n240 = Format Date/Time String(time format string (%c)="%H:%M:%S ") -> (date/time string=w475:string)  [unwired: 2 in]
                n241 = Format Date/Time String(time format string (%c)="%H:%M:%S ") -> (date/time string=w474:string)  [unwired: 2 in]
                n242 = Format Date/Time String(time format string (%c)="%H:%M:%S ") -> (date/time string=w473:string)  [unwired: 2 in]
                n243 = Format Date/Time String(time format string (%c)="%H:%M:%S ") -> (date/time string=w472:string)  [unwired: 2 in]
                n244 = Concatenate Strings(w475, "Program start..." ("string"), "\r\n") -> (w462:string)
                n245 = Concatenate Strings(w474, "Erase success !") -> (w461:string)
                n246 = Concatenate Strings(w473, "Please check COM adaptor, Power Supply and reset unit.", "\r\n") -> (w468:string)
                n247 = Concatenate Strings(w472, "No response, Erase failed !" ("string")) -> (w467:string)
                n248 = Concatenate Strings(w462, w461) -> (w460:string)
                n249 = Concatenate Strings(w468, w467) -> (w466:string)
              }
            }
            n250 = Select(t=w457, s=w459, f=w456) -> (s? t:f=w458:string)
          }
        }
        n251 = Concatenate Strings(w166, "\r\n", w159) -> (w201:string)
        n252 = And(x=w175, y=TRUE) -> (x .and. y?=w207:bool)
        n253 = case shown="True" w130 {
          tunnel: w201 -> [w368 _]
          tunnel: [w367 w369] -> w200
          tunnel: w138 -> [w366 w369]
          frame False {
            n254 = property on="Error List" class="Str"(error in=w366, "Value"=w368) -> (error out=w367:errorcluster)  [unwired: 1 in, 1 out]
          }
          frame True {
          }
        }
        n255 = case shown="True" w207 {
          tunnel: w219 -> [w611 w617]
          tunnel: [w611 w616] -> w195
          tunnel: [w609 w614] -> w177
          tunnel: w173 -> [_ w618]
          tunnel: [FALSE w612] -> w169
          tunnel: w200 -> [w609 w613]
          frame False {
          }
          frame True {
            n256 = for {
              shift-right: [w643] -> _
              shift-left: w618 -> [w654]
              tunnel: w618 -> [_] mode=indexing
              tunnel: [w636] -> w619 mode=indexing
              tunnel: w617 -> [w635]
              tunnel: [w632] -> w616
              tunnel: [w621] -> _ mode=concatenating
              tunnel: [w630] -> w615 mode=indexing
              shift-right: [w631] -> w614
              shift-left: w613 -> [w624]
              tunnel: [w623] -> w612
              tunnel: [w621] -> _ mode=indexing
              i -> [w644]
              stop <- w622 stop-if-true
              n257 = Increment(x=w644) -> (x+1=→"Num of Data packet":i32)
              n258 = Index Array(array=w654) -> (element #1=w653:u8, element #2=w652:u8)  [unwired: 2 in]
              n259 = Join Numbers(hi=w652, lo=w653) -> ((hi.lo)=w626:u16)
              n260 = Add(x=w626, y=u32 3) -> (x+y=w650:u32)
              n261 = property on="stop 6" class="Bool (strict)"() -> ("Value"=w620:bool)  [unwired: 2 in, 2 out]
              n262 = Equal?(x=w626, y=u16 0) -> (x = y?=w647:bool)
              n263 = Multiply(x=w650, y=u32 2) -> (x*y=w648:u32)
              n264 = Or(x=w647, y=w620) -> (x .or. y?=w622:bool)
              n265 = To Long Integer(number=w648) -> (32bit integer=w627:i32)
              n266 = Delete From Array(array=w654, length=w627, index=0) -> (deleted portion=w628:u8[], array with subset deleted=w643:u8[])
              n267 = Array Size(array=w628) -> (size(s)=w640:i32)
              n268 = Divide(x=w640, y=2) -> (x/y=w642:dbl)
              n269 = To Long Integer(number=w642) -> (32bit integer=w639:i32)
              n270 = for {
                N: w639 -> [_]
                tunnel: w628 -> [w887]
                tunnel: [w883] -> w636 mode=indexing
                i -> [w886]
                n271 = Multiply(x=2, y=w886) -> (x*y=w889:i32)
                n272 = Increment(x=w889) -> (x+1=w890:i32)
                n273 = Index Array(array=w887, index #1=w889, index #2=w890) -> (element #1=w885:u8, element #2=w884:u8)
                n274 = Join Numbers(hi=w885, lo=w884) -> ((hi.lo)=w883:u16)
              }
              n275 = Array Size(array=w636) -> (size(s)=w638:i32)
              n276 = Equal?(x=w627, y=6) -> (x = y?=w625:bool)
              n277 = Less Or Equal?(x=w638, y=1027) -> (x <= y?=w633:bool)
              n278 = case shown="False" w620 {
                tunnel: w636 -> [w666 _]
                tunnel: w635 -> [w665 w881]
                tunnel: w633 -> [w664 _]
                tunnel: [w662 w881] -> w632
                tunnel: [w661 w880] -> w631
                tunnel: [w660 u16[] []] -> w630
                tunnel: w625 -> [w659 _]
                tunnel: w624 -> [w658 w880]
                tunnel: [w655 TRUE] -> w623
                tunnel: [w656 bool[] []] -> w621
                frame False {
                  n279 = Or(x=w659, y=w664) -> (x .or. y?=w663:bool)
                  n280 = case shown="True" w663 {
                    tunnel: w658 -> [w671 w799]
                    tunnel: w665 -> [w674 w790]
                    tunnel: [w673 w785] -> w661
                    tunnel: [w672 w801] -> w662
                    tunnel: w666 -> [w669 w800]
                    tunnel: [w670 w797] -> w656
                    tunnel: [w668 w795] -> w660
                    tunnel: w659 -> [_ w794]
                    tunnel: [w667 w784] -> w657
                    frame False {
                      n281 = while {
                        tunnel: w669 -> [_]
                        tunnel: [w676] -> w670 mode=concatenating
                        shift-right: [w696] -> w672
                        shift-left: w674 -> [w697]
                        shift-right: [w679] -> w673
                        shift-left: w671 -> [w695]
                        shift-right: [w688] -> _
                        shift-left: w669 -> [w694]
                        tunnel: [w687] -> w668 mode=indexing
                        tunnel: [w675] -> w667
                        i -> [w686]
                        stop <- w678 stop-if-true
                        n282 = Equal To 0?(x=w686) -> (x = 0?=w685:bool)
                        n283 = Select(t=1027 ("length"), s=w685, f=1024 ("length")) -> (s? t:f=w682:i32)
                        n284 = Delete From Array(array=w694, length=w682, index=0) -> (deleted portion=w689:u16[], array with subset deleted=w688:u16[])
                        n285 = property on="stop 6" class="Bool (strict)"() -> ("Value"=w677:bool)  [unwired: 2 in, 2 out]
                        n286 = Array Size(array=w689) -> (size(s)=w692:i32)
                        n287 = Greater?(x=w692, y=1) -> (0:w690:bool)
                        n288 = Not(x=w690) -> (.not. x?=w680:bool)
                        n289 = Or(x=w680, y=w677) -> (x .or. y?=w678:bool)
                        n290 = case shown="True" w690 {
                          tunnel: w697 -> [w700 w727]
                          tunnel: [w702 w703] -> w679
                          tunnel: [w700 w725] -> w696
                          tunnel: w695 -> [w702 w723]
                          tunnel: [FALSE w718] -> w681
                          tunnel: w689 -> [_ w717]
                          tunnel: [u16 0 ("Numeric") w716] -> w687
                          tunnel: [FALSE w705] -> w675
                          frame False {
                          }
                          frame True {
                            n291 = flat-sequence {
                              tunnel: w723 -> [w734]
                              tunnel: [w738] -> w715
                              tunnel: [w736] -> w719
                              tunnel: w717 -> [w735]
                              tunnel: [w734] -> w724
                              tunnel: [w733] -> w716
                              frame #0 {
                                n292 = for {
                                tunnel: w735 -> [w751] mode=indexing
                                shift-right: [w746] -> w738
                                shift-left: u8[] [] -> [w745]
                                shift-right: [w743] -> w733
                                shift-left: u16 0 -> [w744]
                                i -> [w750]
                                n293 = Split Number(x=w751) -> (hi(x)=w742:u8, lo(x)=w741:u8)
                                n294 = Build Array(w742, w741) -> (w748:u8[])
                                n295 = Compound Arithmetic op=ADD(w744, w742, w741) -> (w743:u16)
                                n296 = Multiply(x=w750, y=2) -> (x*y=w747:i32)
                                n297 = Insert Into Array(array=w745, index=w747, new element=w748) -> (w746:u8[])
                                }
                                "CheckSum DataB" <- w733
                                n298 = Type Cast(type="", x=w733) -> (*(type *) &x=w736:string)
                              }
                            }
                            n299 = Byte Array To String(unsigned byte array=w715) -> (string=w704:string)
                            n300 = VISA Write(VISA resource name=w727, write buffer=w704, error in (no error)=w724) -> (VISA resource name out=w711:refnum<visa-resource-name>, error out=w710:errorcluster)  [unwired: 1 out]
                            n301 = flat-sequence {
                              tunnel: [w732] -> w708
                              tunnel: w710 -> [w731]
                              tunnel: [w731] -> w709
                              frame #0 {
                                n302 = call <vilib>:"High Resolution Relative Seconds.vi"() -> ("relative seconds"=w732:dbl)
                              }
                            }
                            n303 = while {
                              tunnel: w711 -> [w780]
                              tunnel: [w781] -> w728
                              tunnel: [w782] -> w712
                              tunnel: [w775] -> w722
                              tunnel: w709 -> [w771]
                              tunnel: w708 -> [w770]
                              tunnel: [w768] -> w706
                              stop <- w777 stop-if-true
                              n304 = VISA Read(VISA resource name=w780, byte count=u32 1, error in (no error)=w771) -> (VISA resource name out=w781:refnum<visa-resource-name>, read buffer=w775:string, return count=w776:u32, error out=w782:errorcluster)
                              n305 = call <vilib>:"High Resolution Relative Seconds.vi"() -> ("relative seconds"=w772:dbl)
                              n306 = Not Equal?(x=w776, y=u32 0) -> (x != y?=w778:bool)
                              n307 = property on="stop 6" class="Bool (strict)"() -> ("Value"=w769:bool)  [unwired: 2 in, 2 out]
                              n308 = Subtract(x=w772, y=w770) -> (x-y=w773:dbl)
                              n309 = Greater Or Equal?(x=w773, y=1.0) -> (x >= y?=w768:bool)
                              n310 = Compound Arithmetic op=OR(w778, w769, w768) -> (w777:bool)
                              n311 = property on="stop 6" class="Bool (strict)"("Value"=w768) -> ()  [unwired: 2 in, 2 out]
                            }
                            n312 = flat-sequence {
                              tunnel: w712 -> [w730]
                              tunnel: [w730] -> w713
                              tunnel: [w729] -> w714
                              frame #0 {
                                n313 = call <vilib>:"High Resolution Relative Seconds.vi"() -> ("relative seconds"=w729:dbl)
                              }
                            }
                            n314 = while {
                              tunnel: w728 -> [w766]
                              tunnel: [w763] -> w725
                              tunnel: w713 -> [w767]
                              tunnel: [w764] -> w726
                              tunnel: [w758] -> w721
                              tunnel: w714 -> [w754]
                              tunnel: [w752] -> w707
                              stop <- w759 stop-if-true
                              n315 = VISA Read(VISA resource name=w766, byte count=u32 1, error in (no error)=w767) -> (VISA resource name out=w763:refnum<visa-resource-name>, read buffer=w758:string, return count=w760:u32, error out=w764:errorcluster)
                              n316 = call <vilib>:"High Resolution Relative Seconds.vi"() -> ("relative seconds"=w757:dbl)
                              n317 = Not Equal?(x=w760, y=u32 0) -> (x != y?=w762:bool)
                              n318 = Subtract(x=w757, y=w754) -> (x-y=w756:dbl)
                              n319 = property on="stop 6" class="Bool (strict)"() -> ("Value"=w753:bool)  [unwired: 2 in, 2 out]
                              n320 = Greater Or Equal?(x=w756, y=1.0) -> (x >= y?=w752:bool)
                              n321 = Compound Arithmetic op=OR(w762, w753, w752) -> (w759:bool)
                              n322 = property on="stop 6" class="Bool (strict)"("Value"=w752) -> ()  [unwired: 2 in, 2 out]
                            }
                            n323 = Or(x=w707, y=w706) -> (x .or. y?=w705:bool)
                            n324 = Concatenate Strings(w721, w722) -> (w720:string)
                            n325 = call "Time Delay4"("error in (no error)"=w726) -> ("error out"=w703:errorcluster)  [unwired: 10 in]
                            n326 = Equal?(x=w719, y=w720) -> (x = y?=w718:bool)
                          }
                        }
                        n327 = property on="stop 6" class="Bool (strict)"("Value"=w675) -> ()  [unwired: 2 in, 2 out]
                        n328 = Build Array(w681) -> (w676:bool[])
                      }
                    }
                    frame True {
                      n329 = flat-sequence {
                        tunnel: w799 -> [w860]
                        tunnel: [w864] -> w792
                        tunnel: [w862] -> w793
                        tunnel: w800 -> [w861]
                        tunnel: [w860] -> w791
                        tunnel: [w859] -> w796
                        frame #0 {
                          n330 = for {
                            tunnel: w861 -> [w877] mode=indexing
                            shift-right: [w872] -> w864
                            shift-left: u8[] [] -> [w871]
                            shift-right: [w869] -> w859
                            shift-left: u16 0 -> [w870]
                            i -> [w876]
                            n331 = Split Number(x=w877) -> (hi(x)=w868:u8, lo(x)=w867:u8)
                            n332 = Build Array(w868, w867) -> (w874:u8[])
                            n333 = Compound Arithmetic op=ADD(w870, w868, w867) -> (w869:u16)
                            n334 = Multiply(x=w876, y=2) -> (x*y=w873:i32)
                            n335 = Insert Into Array(array=w871, index=w873, new element=w874) -> (w872:u8[])
                          }
                          "CheckSum Data" <- w859
                          n336 = Type Cast(type="", x=w859) -> (*(type *) &x=w862:string)
                        }
                      }
                      n337 = Build Array(w796) -> (w795:u16[])
                      n338 = Byte Array To String(unsigned byte array=w792) -> (string=w787:string)
                      n339 = VISA Write(VISA resource name=w790, write buffer=w787, error in (no error)=w791) -> (VISA resource name out=w789:refnum<visa-resource-name>, error out=w788:errorcluster)  [unwired: 1 out]
                      n340 = case shown="False" w794 {
                        tunnel: w789 -> [w817 w857]
                        tunnel: w788 -> [w810 w856]
                        tunnel: [w802 w856] -> w785
                        tunnel: [w815 w857] -> w801
                        tunnel: [w812 "\u0000\u0000"] -> w798
                        tunnel: [w803 FALSE] -> w784
                        frame False {
                          n341 = flat-sequence {
                            tunnel: [w822] -> w811
                            tunnel: w810 -> [w821]
                            tunnel: [w821] -> w809
                            frame #0 {
                              n342 = call <vilib>:"High Resolution Relative Seconds.vi"() -> ("relative seconds"=w822:dbl)
                            }
                          }
                          n343 = while {
                            tunnel: w817 -> [w851]
                            tunnel: [w852] -> w818
                            tunnel: w809 -> [w850]
                            tunnel: [w853] -> w808
                            tunnel: [w845] -> w814
                            tunnel: w811 -> [w843]
                            tunnel: [w839] -> w804
                            stop <- w847 stop-if-true
                            n344 = VISA Read(VISA resource name=w851, byte count=u32 1, error in (no error)=w850) -> (VISA resource name out=w852:refnum<visa-resource-name>, read buffer=w845:string, return count=w846:u32, error out=w853:errorcluster)
                            n345 = call <vilib>:"High Resolution Relative Seconds.vi"() -> ("relative seconds"=w844:dbl)
                            n346 = Not Equal?(x=w846, y=u32 0) -> (x != y?=w848:bool)
                            n347 = Subtract(x=w844, y=w843) -> (x-y=w842:dbl)
                            n348 = property on="stop 6" class="Bool (strict)"() -> ("Value"=w840:bool)  [unwired: 2 in, 2 out]
                            n349 = Greater Or Equal?(x=w842, y=1.0) -> (x >= y?=w839:bool)
                            n350 = Compound Arithmetic op=OR(w848, w840, w839) -> (w847:bool)
                            n351 = property on="stop 6" class="Bool (strict)"("Value"=w839) -> ()  [unwired: 2 in, 2 out]
                          }
                          n352 = flat-sequence {
                            tunnel: w808 -> [w820]
                            tunnel: [w820] -> w807
                            tunnel: [w819] -> w806
                            frame #0 {
                              n353 = call <vilib>:"High Resolution Relative Seconds.vi"() -> ("relative seconds"=w819:dbl)
                            }
                          }
                          n354 = while {
                            tunnel: w818 -> [w837]
                            tunnel: [w834] -> w815
                            tunnel: w807 -> [w838]
                            tunnel: [w835] -> w816
                            tunnel: [w829] -> w813
                            tunnel: w806 -> [w825]
                            tunnel: [w823] -> w805
                            stop <- w830 stop-if-true
                            n355 = VISA Read(VISA resource name=w837, byte count=u32 1, error in (no error)=w838) -> (VISA resource name out=w834:refnum<visa-resource-name>, read buffer=w829:string, return count=w831:u32, error out=w835:errorcluster)
                            n356 = call <vilib>:"High Resolution Relative Seconds.vi"() -> ("relative seconds"=w826:dbl)
                            n357 = Not Equal?(x=w831, y=u32 0) -> (x != y?=w833:bool)
                            n358 = Subtract(x=w826, y=w825) -> (x-y=w827:dbl)
                            n359 = property on="stop 6" class="Bool (strict)"() -> ("Value"=w824:bool)  [unwired: 2 in, 2 out]
                            n360 = Greater Or Equal?(x=w827, y=1.0) -> (x >= y?=w823:bool)
                            n361 = Compound Arithmetic op=OR(w833, w824, w823) -> (w830:bool)
                            n362 = property on="stop 6" class="Bool (strict)"("Value"=w823) -> ()  [unwired: 2 in, 2 out]
                          }
                          n363 = Or(x=w805, y=w804) -> (x .or. y?=w803:bool)
                          n364 = Concatenate Strings(w813, w814) -> (w812:string)
                          n365 = call "Time Delay5"("error in (no error)"=w816) -> ("error out"=w802:errorcluster)  [unwired: 10 in]
                        }
                        frame True {
                        }
                      }
                      n366 = property on="stop 6" class="Bool (strict)"("Value"=w784) -> ()  [unwired: 2 in, 2 out]
                      n367 = Equal?(x=w793, y=w798) -> (x = y?=w786:bool)
                      n368 = Build Array(w786) -> (w797:bool[])
                    }
                  }
                  n369 = Not(x=w657) -> (.not. x?=w655:bool)
                }
                frame True {
                }
              }
            }
            "Array 3" <- w619
            "CheckSumArray" <- w615
          }
        }
        n370 = call <vilib>:"Clear Errors.vi"("error in (no error)"=w177) -> ("error out"=w176:errorcluster)  [unwired: 5 in, 1 out]
        n371 = property on="stop 6" class="Bool (strict)"(error in=w176) -> (error out=w128:errorcluster, "Value"=w133:bool)  [unwired: 1 in, 1 out]
        n372 = property on="Error List" class="Str"(error in=w128) -> (error out=w137:errorcluster, "Value"=w162:string)  [unwired: 1 in, 1 out]
        n373 = case shown="True" w169 {
          tunnel: ["" w433] -> w165
          tunnel: w133 -> [_ w430]
          tunnel: [TRUE ("Value") w430] -> w174
          tunnel: w137 -> [_ w429]
          frame False {
          }
          frame True {
            n374 = flat-sequence {
              tunnel: [w440] -> w432
              tunnel: [w434] -> w431
              tunnel: w429 -> [_]
              frame #0 {
                n375 = Format Date/Time String(time format string (%c)="%H:%M:%S ") -> (date/time string=w449:string)  [unwired: 2 in]
                n376 = Format Date/Time String(time format string (%c)="%H:%M:%S ") -> (date/time string=w448:string)  [unwired: 2 in]
                n377 = Format Date/Time String(time format string (%c)="%H:%M:%S ") -> (date/time string=w447:string)  [unwired: 2 in]
                n378 = Format Date/Time String(time format string (%c)="%H:%M:%S ") -> (date/time string=w446:string)  [unwired: 2 in]
                n379 = Concatenate Strings(w449, "Program failed !" ("string"), "\r\n") -> (w436:string)
                n380 = Concatenate Strings(w448, "Please check COM adaptor or try a different baudrate.") -> (w435:string)
                n381 = Concatenate Strings(w447, "Getting Driver version...", "\r\n") -> (w442:string)
                n382 = Concatenate Strings(w446, "Program success !" ("string")) -> (w441:string)
                n383 = Concatenate Strings(w436, w435) -> (w434:string)
                n384 = Concatenate Strings(w442, w441) -> (w440:string)
              }
            }
            n385 = Select(t=w431, s=w430, f=w432) -> (s? t:f=w433:string)
          }
        }
        n386 = Concatenate Strings(w165, "\r\n", w162) -> (w199:string)
        n387 = case shown="False" w133 {
          tunnel: w199 -> [w364 _]
          tunnel: [w363 w365] -> w183
          tunnel: w137 -> [w362 w365]
          frame False {
            n388 = property on="Error List" class="Str"(error in=w362, "Value"=w364) -> (error out=w363:errorcluster)  [unwired: 1 in, 1 out]
          }
          frame True {
          }
        }
        n389 = VISA Clear(VISA resource name=w195, error in (no error)=w183) -> (VISA resource name out=w184:refnum<visa-resource-name>, error out=w182:errorcluster)
        n390 = case shown="False" w133 {
          tunnel: w182 -> [w485 w532]
          tunnel: w184 -> [w484 _]
          tunnel: [w481 w532] -> w187
          tunnel: [w483 0 ("D Int out")] -> w193
          tunnel: [w482 FALSE] -> w192
          frame False {
            n391 = case shown="True" TRUE {
              tunnel: [w496 w501] -> w487
              tunnel: [w494 w500] -> w486
              tunnel: w485 -> [w495 w498]
              tunnel: w484 -> [w496 w497]
              frame False {
                n392 = call "Time Delay3"("error in (no error)"=w495) -> ("error out"=w494:errorcluster)  [unwired: 10 in]
              }
              frame True {
                w509 = u16 0 items=["None", "XON/XOFF", "RTS/CTS", "XON/XOFF & RTS/CTS", "DTR/DSR", "XON/XOFF & DTR/DSR"] ("flow control (0:none)")
                w508 = u16 10 items=["1.0"=10, "1.5"=15, "2.0"=20] ("stop bits (10: 1 bit)")
                w510 = T4 1073684533 items=["Service Request"=1073684491, "Trigger"=3221168138, "Clear"=1073684493, "VXI Signal"=1073684512, "VXI/VME Interrupt"=3221168161, "VXI/VME Sysfail"=1073684509, "VXI/VME Sysreset"=1073684510, "GPIB CIC"=1073684498, "GPIB Talk"=1073684499, "GPIB Listen"=1073684500, "PXI Interrupt"=1073684514, "Serial Break"=1073684515, "Serial TermChar"=1073684516, "Serial CTS"=1073684521, "Serial DSR"=1073684522, "Serial DCD"=1073684524, "Serial RI"=1073684526, "Serial Character"=1073684533, "USB Interrupt"=1073684535, "All Enabled"=1073709055] ("Event Type")
                n393 = call-poly "VISA Configure Serial Port"("VISA resource name"=w497, "timeout (10sec)"=u32 200, "Enable Termination\nChar (T)"=FALSE ("Enable Termination\nChar (T)"), "baud rate (9600)"=u32 230400, "data bits (8)"=u16 8, "parity (0:none)"=enum16{"None", "Odd", "Even", "Mark", "Space"}."None", "error in (no error)"=w498, "stop bits (10: 1 bit)"=w508, "flow control (0:none)"=w509) -> ("VISA resource name out"=w502:refnum<visa-resource-name>, "error out"=w503:errorcluster)  [unwired: 5 in]
                n394 = VISA Enable Event(8:w503, 10:w510, 11:w502) -> (0:w500:errorcluster, 3:w501:refnum<visa-resource-name>)  [unwired: 1 in]
              }
            }
            n395 = Byte Array To String(unsigned byte array=u8[] [73, 93, 62, 192, 16, 48, 0] ("output array")) -> (string=w491:string)
            n396 = VISA Write(VISA resource name=w487, write buffer=w491, error in (no error)=w486) -> (VISA resource name out=w493:refnum<visa-resource-name>, error out=w490:errorcluster)  [unwired: 1 out]
            n397 = flat-sequence {
              tunnel: w490 -> [w512]
              tunnel: [w512] -> w489
              tunnel: [w511] -> w488
              frame #0 {
                n398 = call <vilib>:"High Resolution Relative Seconds.vi"() -> ("relative seconds"=w511:dbl)
              }
            }
            n399 = while {
              tunnel: w489 -> [w529]
              tunnel: [w527] -> w481
              tunnel: w493 -> [w528]
              tunnel: w488 -> [w520]
              tunnel: [w515] -> w483
              tunnel: [w514] -> w482
              stop <- w517 stop-if-true
              n400 = call <vilib>:"High Resolution Relative Seconds.vi"() -> ("relative seconds"=w521:dbl)
              n401 = VISA Read(VISA resource name=w528, byte count=u32 11, error in (no error)=w529) -> (read buffer=w525:string, return count=w522:u32, error out=w527:errorcluster)  [unwired: 1 out]
              n402 = Subtract(x=w521, y=w520) -> (x-y=w518:dbl)
              n403 = String To Byte Array(string=w525) -> (unsigned byte array=w524:u8[])
              n404 = Not Equal To 0?(x=w522) -> (x != 0?=w514:bool)
              n405 = Greater Or Equal?(x=w518, y=3.0) -> (x >= y?=w516:bool)
              n406 = property on="stop 6" class="Bool (strict)"() -> ("Value"=w513:bool)  [unwired: 2 in, 2 out]
              n407 = call "Data_Convert.vi"("Data Type"=u8 0, "Array"=w524) -> ("D Int out"=w515:i32)  [unwired: 2 out]
              n408 = Compound Arithmetic op=OR(w513, w514, w516) -> (w517:bool)
            }
          }
          frame True {
          }
        }
        n409 = call <vilib>:"Clear Errors.vi"("error in (no error)"=w187) -> ("error out"=w185:errorcluster)  [unwired: 5 in, 1 out]
        n410 = property on="Error List" class="Str"(error in=w185) -> (error out=w136:errorcluster, "Value"=w163:string)  [unwired: 1 in, 1 out]
        n411 = case shown="False" w174 {
          tunnel: w193 -> [w419 _]
          tunnel: w192 -> [w418 _]
          tunnel: [w413 "" ("f")] -> w135
          tunnel: w136 -> [w415 _]
          frame False {
            n412 = Format Into String(w419) -> (resulting string=w420:string)  [unwired: 3 in, 1 out]
            n413 = flat-sequence {
              tunnel: w414 -> [w423]
              tunnel: w415 -> [_]
              tunnel: [w422] -> w413
              frame #0 {
                n414 = Format Date/Time String(time format string (%c)="%H:%M:%S ") -> (date/time string=w424:string)  [unwired: 2 in]
                n415 = Concatenate Strings(w424, w423) -> (w422:string)
              }
            }
            n416 = Concatenate Strings("Driver Version: " ("string"), w420) -> (w416:string)
            n417 = Select(t=w416, s=w418, f="Getting Driver version failed !") -> (s? t:f=w414:string)
          }
          frame True {
          }
        }
        n418 = Concatenate Strings(w135, "\r\n", w163) -> (w191:string)
        n419 = case shown="False" w133 {
          tunnel: [w360 w361] -> w194
          tunnel: w191 -> [w359 _]
          tunnel: w136 -> [w358 w361]
          frame False {
            n420 = property on="Error List" class="Str"(error in=w358, "Value"=w359) -> (error out=w360:errorcluster)  [unwired: 1 in, 1 out]
          }
          frame True {
          }
        }
        n421 = VISA Close(VISA resource name=w184, error in (no error)=w194) -> (error out=w170:errorcluster)
      }
    }
    n422 = Or(x="stop 6", y=FALSE) -> (x .or. y?=w62:bool)
    n423 = call <vilib>:"Clear Errors.vi"("error in (no error)"=w96) -> ("error out"=w86:errorcluster)  [unwired: 5 in, 1 out]
    n424 = property on="Next Button" class="Bool (strict)"(error in=w86, "Value"=w84, "Blinking"=w84) -> (error out=w95:errorcluster)  [unwired: 1 in, 1 out]
  }
  "error out" <- w30
